vi "FPGA_AnalogTriggerConvertSourceToFPGA.vi"(8 "error in (no error)":errorcluster, 11 "AnalogTriggerSource":T2={"Channel"=enum."AI 1", "Averaged"=FALSE, "Filter"=FALSE}) -> (0 "error out":errorcluster, 3 "FPGASourceType":T1)   [LabVIEW 2017]
uses:
  <vilib>/Rock Robotics/SystemInterfaces/AnalogTrigger/FPGA_AnalogTriggerSource.ctl
  <vilib>/Rock Robotics/SystemInterfaces/AI/FPGA_AIChannel.ctl
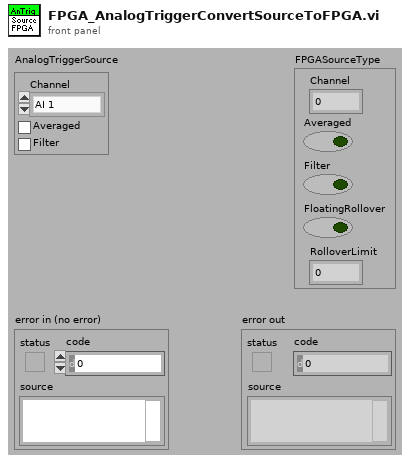
[diagram p1: front panel]
types:
  T1 = cluster{"Channel":fxp<+,3,3>, "Averaged":bool, "Filter":bool, "FloatingRollover":bool, "RolloverLimit":fxp<+/-,8,12>}
  T2 = typedef "FPGA_AnalogTriggerSource.ctl" = cluster{"Channel":T3, "Averaged":bool, "Filter":bool}
  T3 = typedef "FPGA_AIChannel.ctl" = enum8{"AI 0", "AI 1", "AI 2", "AI 3", "AI MXP 0", "AI MXP 1", "AI MXP 2", "AI MXP 3", "Invalid"}
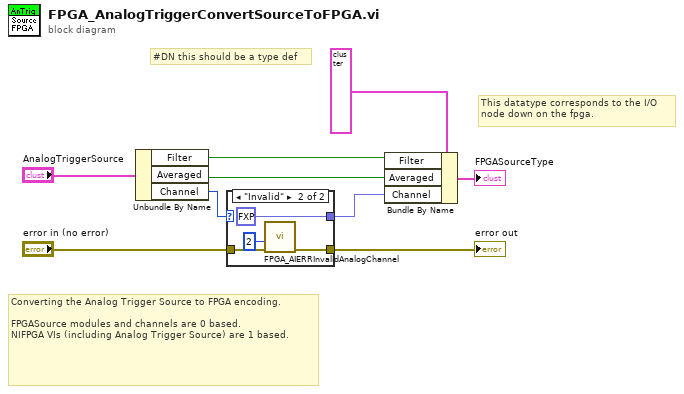
[diagram p0: block diagram]
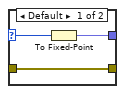
[diagram p2: hidden frame]
diagram:
  # "#DN this should be a type def"
  # "This datatype corresponds to the I/O\nnode down on the fpga."
  # "Converting the Analog Trigger Source to FPGA encoding.\n\nFPGASource modules and channels are 0 based.\nNIFPGA VIs (including Analog Trigger Source) are 1 based."
  n1 = Unbundle By Name("AnalogTriggerSource") -> ("Filter"=w7:bool, "Averaged"=w6:bool, "Channel"=w5:T3)
  n2 = case shown="\"Invalid\"" w5 {
    selector: w5 -> [w12 _]
    tunnel: [w10 w14] -> w3
    tunnel: [w11 fxp<+,3,3> 0.0 ("Channel")] -> w4
    tunnel: "error in (no error)" -> [w10 w15]
    frame Default {
      n3 = To Fixed-Point(number=w12) -> (fixed-point=w11:fxp<+,3,3>)  [unwired: 1 out]
    }
    frame "Invalid" {
      n4 = call <vilib>:"FPGA_AIERRInvalidAnalogChannel.vi"("error in (no error)"=w15, "Additional Depth"=2) -> ("error out"=w14:errorcluster)  [unwired: 9 in]
    }
  }
  "error out" <- w3
  n5 = Bundle By Name(cluster=T1 {"Channel"=0.0, "Averaged"=FALSE, "Filter"=FALSE, "FloatingRollover"=FALSE, "RolloverLimit"=0.0} ("AnalogTrigger0.SourceSelect"), "Filter"=w7, "Averaged"=w6, "Channel"=w4) -> (→"FPGASourceType":T1)
